vi "2100_Test_Set State_Measure Resistance_SH3T_Rfree_w Config.vi"(0 "Semiconductor Module Context":T7, 1 "Script_Info":T3={"Script Name"="WalkingState", "All_Scripts"=[]}, 4 "Instrument_Pins":T6={"SMU_Pins"=["RF1", "RF2", "RF3", "RF4"], "HSDIO_Pins"=["CLK", "SDA"]}, 5 "Error In":errorcluster, 6 "USID":T4 max=15, 7 "Master_Register_Data_Array_In":T1 {"Address" format="%.0x"}, 8 "current range":dbl format="%#_6p", 10 "current level":dbl=1e-05 format="%#_13p", 11 "Reg_Map_and_Bit_Name":T5={"Reg_Map_Bit_Name"="", "Reg_Map"=[["Reg Addr(0x00)", "7", "6", "5", "4", "3", "2", "1", "0"], ["0", "SPARE", "RF3_SH", "RF2_SH", "RF1_SH", "SPARE", "RF3_RFC", "RF2_RFC", "RF1_RFC"], ["1", "SPARE[7:0]", "", "", "", "", "", "", ""], ["2", "VVAR_EN", "LCM_EN", "RFC_SH", "SPARE", "VARACTOR[3:0]", "", "", ""], ["3", "SW_CTRL1_VIRTUAL[7:0]", "", "", "", "", "", "", ""], ["4", "SW_CTRL1_SWAP", "SW_CTRL1_RBSHIFT[2:0]", "", "", "SW_CTRL1_VSID[3:0]", "", "", ""], ["5", "REG_00_VIRTUAL_MASK[7:0]", "", "", "", "", "", "", ""], ["6", "LOCK_STATUS[1:0]", "", "CLK_DITHER", "FUSES_BURNED", "CLK_IDAC_CAL[3:0]", "", "", ""], ["7", "SPARE[2:0]", "", "", "ODFT_TRIM[4:0]", "", "", "", ""], ["8", "SPARE[2:0]", "", "", "HV_TRIM[4:0]", "", "", "", ""], ["9", "TEST_MUX[2:0]", "", "", "SPARE[1:0]", "", "MEMS_BG_TC[1:0]", "", "MEMSCP_RCM"], ["A", "CP_BOOST_OVRD_EN", "SPARE[2:0]", "", "", "PS_OFF_TIMER[1:0]", "", "PS_ON_TIMER[1:0]", ""], ["0", "", "", "", "", "", "", "", ""], ["D", "Reserved[1:0]", "", "WD_HI_EVENT_CNT[5:0]", "", "", "", "", ""], ["E", "VERSION_ID[7:0]", "", "", "", "", "", "", ""], ["F", "Reserved", "COUNT_200_LSB[6:0]", "", "", "", "", "", ""], ["10", "CLK_DIV2_EN", "Spare", "ODFT_EN", "HV_HYST[4:0]", "", "", "", ""], ["0", "", "", "", "", "", "", "", ""], ["12", "SHORT_FUSE", "FUSE_BURN", "STROBE_EN", "VIO_OK", "RTH[1:0]", "", "FUSE_LOAD_MAN_EN", "FUSE_LOAD"], ["13", "RR_ACK_EN", "Reserved", "ACK_POSITION[1:0]", "", "SuBUS_DRIVE_STRENGTH[3:0]", "", "", ""], ["14", "TM_IO_EN", "TM_IO_SEL", "SuBUS_OVS[1:0]", "", "Reserved[3:0]", "", "", ""], ["15", "Reserved[4:0]", "", "", "", "", "SuBUS_VERSION_PRESENT", "SuBUS_VOLTAGE", "SuBUS_FLAVOR_DEF"], ["16", "PROG_STROBE1_DUR[7:0]", "", "", "", "", "", "", ""], ["17", "PROG_STROBE0_DUR[7:0]", "", "", "", "", "", "", ""], ["18", "Reserved[2:0]", "", "", "EFUSE_SINGLE_ADDR_SEL[4:0]", "", "", "", ""], ["19", "POLL_ADR[4:0]", "", "", "", "", "POLL_BC[2:0]", "", ""], ["1A", "SOFTWARE_RESET", "Reserved[6:0]", "", "", "", "", "", ""], ["1B", "Reserved[7:0]", "", "", "", "", "", "", ""], ["1C", "PWR_MODE_1", "PWR_MODE_0", "TRIGGER_MASK[2:0]", "", "", "TRIGGER[2:0]", "", ""], ["1D", "PRODUCT_ID[7:0]", "", "", "", "", "", "", ""], ["1E", "MANUFACTURER_ID_LSB[7:0]", "", "", "", "", "", "", ""], ["1F", "MANUFACTURER_ID_MSB[3:0]", "", "", "", "USID[3:0]", "", "", ""]]}, 12 "R_Guardian":dbl[](array[numeric])) -> (15 "Master_Register_Data_Array_Out":T1 {"Address" format="%.0x"}, 19 "Error Out":errorcluster)   [LabVIEW 2013]
uses:
  Controls/USID.ctl
  <vilib>/NI_TestStand_SemiconductorModule/NI_TestStand_Semiconductor_Module.lvlibp/PinMap/General/SemiconductorModuleContext.ctl
  Controls/Master_Reg_Data_Array.ctl
  Controls/Reg_Address_Data.ctl
  <vilib>/NI_TestStand_SemiconductorModule/NI_TestStand_Semiconductor_Module.lvlibp/PinMap/General/Publish/PublishDataDoubleFunctionalTest.vi
  <vilib>/NI_TestStand_SemiconductorModule/NI_TestStand_Semiconductor_Module.lvlibp
panel:
  out "Data_Names":string[](array[string])
  out "Logged_Data":dbl[](array[numeric]) format="%#_6p"
  out "R_Measurements":dbl[][](array[numeric]) format="%#_6p"
  in  "Tab Control":enum32{"Test Info", "Instrument Settings"}(tab)
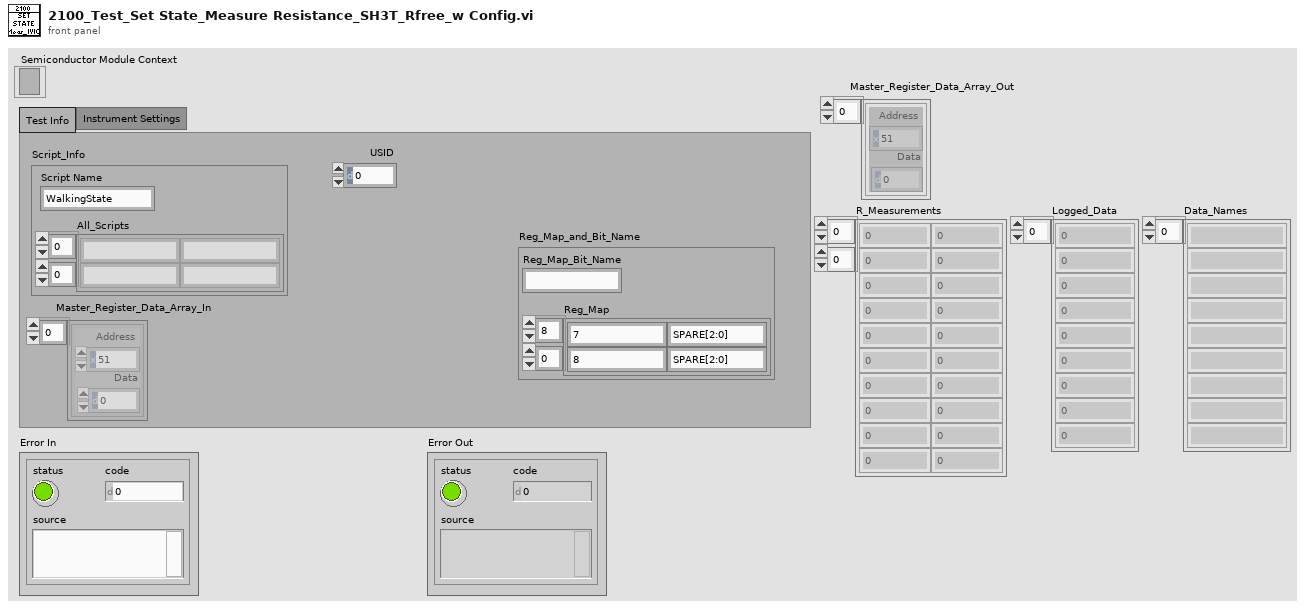
[diagram p1: front panel]
types:
  T1 = typedef "Master_Reg_Data_Array.ctl" = T2[]
  T2 = typedef "Reg_Address_Data.ctl" = cluster{"Address":u8, "Data":u8}
  T3 = cluster{"Script Name":string, "All_Scripts":string[][]}
  T4 = typedef "USID.ctl" = u8
  T5 = cluster{"Reg_Map_Bit_Name":string, "Reg_Map":string[][]}
  T6 = cluster{"SMU_Pins":string[], "HSDIO_Pins":string[]}
  T7 = typedef "NI_TestStand_Semiconductor_Module.lvlibp/SemiconductorModuleContext.ctl" = refnum<k7>
  T8 = typedef "Script Functions_Array.ctl" = enum16{"Reg_Write", "Bit_Write", "Delay", "Read", "Measure"}[]
  T9 = enum16{"Reg_Write", "Bit_Write", "Delay", "Read", "Measure"}
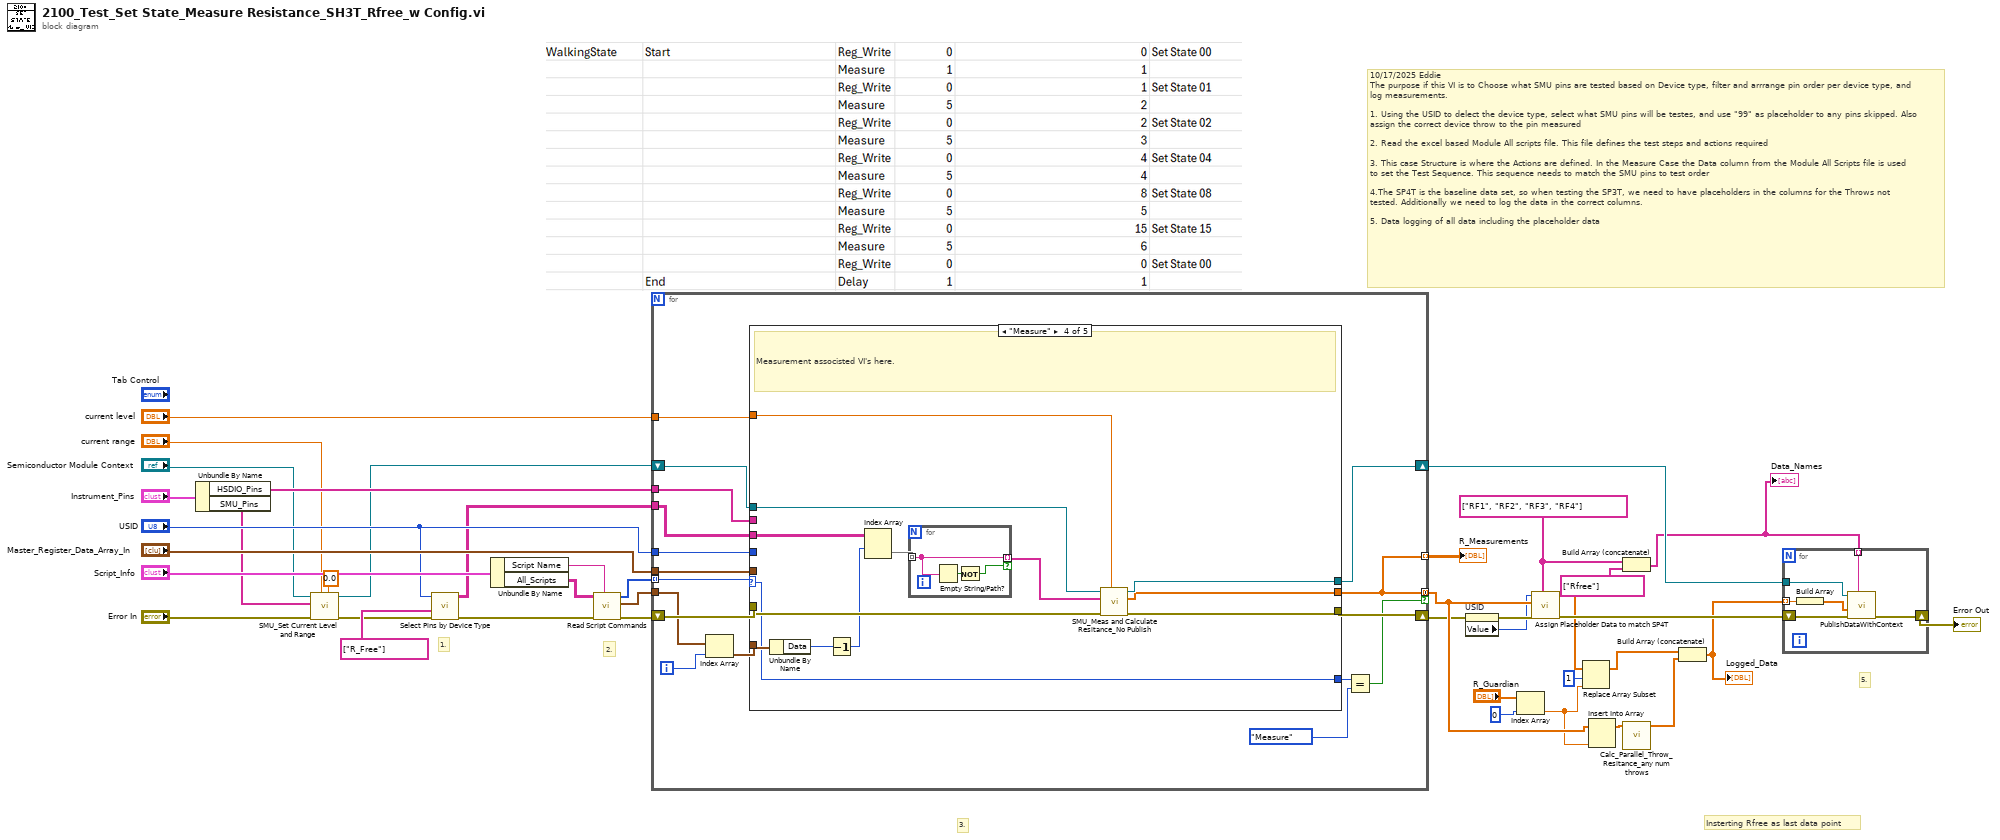
[diagram p0: block diagram]
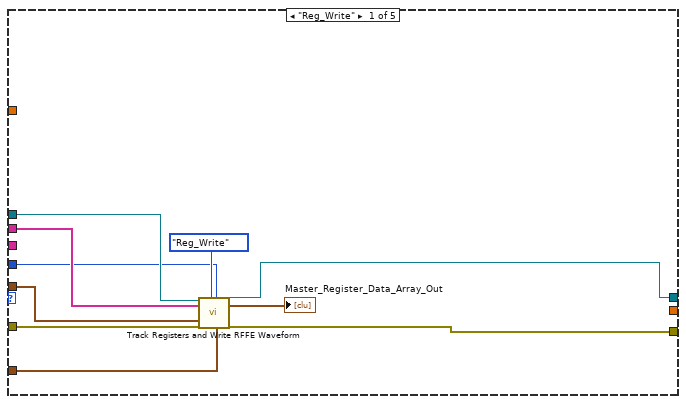
[diagram p2: hidden frame]
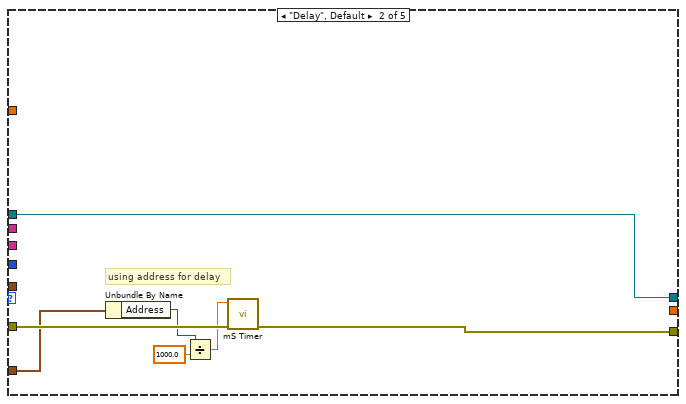
[diagram p3: hidden frame]
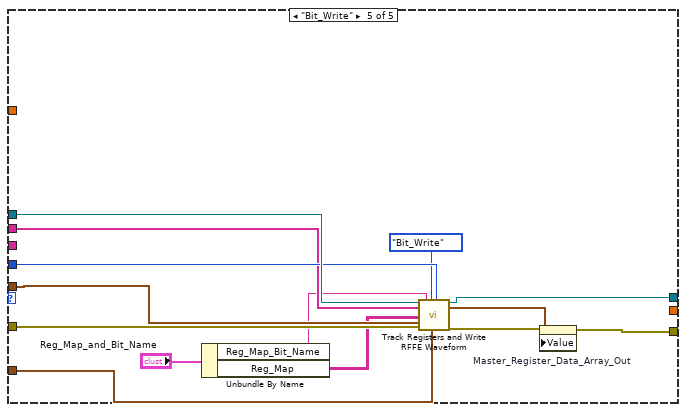
[diagram p5: hidden frame]
diagram:
  w24 = string[] ["RF1", "RF2", "RF3", "RF4"] ("SP4T_Pins")
  # "Insterting Rfree as last data point"
  # "10/17/2025 Eddie \nThe purpose if this VI is to Choose what SMU pins are tested based on Device type, filter and arrrange pin order per device type, and log measurements.\n\n1. Using the USID to delect the device type, select what SMU pins will be testes, and use \"99\" as placeholder to any pins skipped. Also assign the correct device throw to the pin measured\n\n2. Read the excel based Module All scripts file. This file defines the test steps and actions required\n\n3. This case Structure is where the Actions are defined. In the Measure Case the Data column from the Module All Scripts file is used to set the Test Sequence. This sequence needs to match the SMU pins to test order\n\n4.The SP4T is the baseline data set, so when testing the SP3T, we need to have placeholders in the columns for the Throws not tested. Additionally we need to log the data in the correct columns.\n\n5. Data logging of all data including the placeholder data"
  # "5."
  # "3."
  # "2."
  # "1."
  n1 = Unbundle By Name("Instrument_Pins") -> ("HSDIO_Pins"=w35:string[], "SMU_Pins"=w6:string[])
  n2 = call "SMU_Set Current Level and Range.vi"("current level"=0.0, "current range"="current range", "error in (no error)"="Error In", "Pins"=w6, "Semiconductor Module Context"="Semiconductor Module Context") -> ("error out"=w7:errorcluster, "Semiconductor Module Context Out"=w4:T7)  [unwired: 5 in]
  n3 = call "Select Pins by Device Type.vi"("error in (no error)"=w7, "Publishable IDs"=string[] ["R_Free"], "USID"="USID") -> ("error out"=w31:errorcluster, "Pins to Test"=w29:string[][])  [unwired: 7 in]
  n4 = Unbundle By Name("Script_Info") -> ("Script Name"=w32:string, "All_Scripts"=w33:string[][])
  n5 = call "Read Script Commands.vi"("Test Name"=w32, "Error In"=w31, "All_Scripts"=w33) -> ("Error Out"=w39:errorcluster, "Script_Data"=w40:T2[], "Script_Functions"=w41:T8)  [unwired: 5 in, 1 out]
  n6 = for {
    tunnel: "USID" -> [w52]
    tunnel: w41 -> [w51] mode=indexing
    tunnel: w40 -> [w55]
    tunnel: w35 -> [w56]
    shift-right: [w49] -> w11
    shift-left: w39 -> [w58]
    tunnel: "Master_Register_Data_Array_In" -> [w53]
    tunnel: [w47] -> w37 mode=indexing
    tunnel: w29 -> [w48]
    tunnel: [w47] -> w16 mode=concatenating if=w43
    shift-right: [w46] -> w27
    shift-left: w4 -> [w57]
    tunnel: "current level" -> [w42]
    i -> [w50]
    n7 = Index Array(array=w55, index=w50) -> (element=w54:T2)
    n8 = case shown="\"Measure\"" w51 {
      selector: w51 -> [_ _ _ w80 _]
      tunnel: w54 -> [w63 w74 _ w87 w94]
      tunnel: w58 -> [w68 w75 w77 w89 w107]
      tunnel: w52 -> [w60 _ _ _ w101]
      tunnel: w57 -> [w66 w69 w76 w88 w102]
      tunnel: w56 -> [w65 _ _ _ w99]
      tunnel: [w67 w73 w77 w90 w105] -> w49
      tunnel: w53 -> [w62 _ _ _ w98]
      tunnel: [_ _ _ w81 _] -> w47
      tunnel: w48 -> [_ _ _ w86 _]
      tunnel: [w59 w69 w76 w85 w103] -> w46
      tunnel: [_ _ _ w80 _] -> w45
      tunnel: w42 -> [_ _ _ w78 _]
      frame "Reg_Write" {
        n9 = call "Track Registers and Write RFFE Waveform.vi"("Semiconductor Module Context"=w66, "Pins"=w65, "Master_Register_Data_Array_In"=w62, "Error In"=w68, "Script_Functions"=enum16{"Reg_Write", "Bit_Write"}."Reg_Write", "USID"=w60, "Reg_Address_Data"=w63) -> ("Semiconductor Module Context Out"=w59:T7, "Master_Register_Data_Array_Out"=→"Master_Register_Data_Array_Out":T1, "Error Out"=w67:errorcluster)  [unwired: 10 in]
      }
      frame "Delay", Default {
        # "using address for delay"
        n10 = Unbundle By Name(w74) -> ("Address"=w71:u8)
        n11 = Divide(x=w71, y=1000.0) -> (x/y=w70:dbl)
        n12 = call "mS Timer.vi"("Error In"=w75, "Delay(S)"=w70) -> ("Error Out"=w73:errorcluster)  [unwired: 9 in]
      }
      frame "Read" {
        # "Future Dev Code"
      }
      frame "Measure" {
        # "Measurement associsted VI's here."
        n13 = Unbundle By Name(w87) -> ("Data"=w83:u8)
        n14 = Decrement(x=w83) -> (x-1=w82:u8)
        n15 = Index Array(array=w86, index (row)=w82) -> (element=w84:string[])  [unwired: 1 in]
        n16 = for {
          tunnel: w84 -> [w93] mode=indexing
          tunnel: [w93] -> w79 mode=indexing if=w91
          n17 = Empty String/Path?(string/path=w93) -> (empty?=w92:bool)
          n18 = Not(x=w92) -> (.not. x?=w91:bool)
        }
        n19 = call "SMU_Meas and Calculate Resitance_No Publish.vi"("Current  Level"=w78, "error in (no error)"=w89, "Pins"=w79, "Semiconductor Module Context"=w88) -> ("error Out"=w90:errorcluster, "R Array"=w81:dbl[], "Semiconductor Module Context Out"=w85:T7)  [unwired: 4 in, 1 out]
      }
      frame "Bit_Write" {
        n20 = Unbundle By Name("Reg_Map_and_Bit_Name") -> ("Reg_Map_Bit_Name"=w96:string, "Reg_Map"=w95:string[][])
        n21 = call "Track Registers and Write RFFE Waveform.vi"("Semiconductor Module Context"=w102, "Pins"=w99, "Reg_Map"=w95, "Master_Register_Data_Array_In"=w98, "Error In"=w107, "Reg_Map_Bit_Name"=w96, "Script_Functions"=enum16{"Reg_Write", "Bit_Write"}."Bit_Write", "USID"=w101, "Reg_Address_Data"=w94) -> ("Semiconductor Module Context Out"=w103:T7, "Master_Register_Data_Array_Out"=w104:T1, "Error Out"=w106:errorcluster)  [unwired: 8 in]
        n22 = property on="Master_Register_Data_Array_Out" class="Arr (strict)"(error in=w106, "Value"=w104) -> (error out=w105:errorcluster)  [unwired: 1 in, 1 out]
      }
    }
    n23 = Equal?(x=w45, y=T9."Measure" ("Enum")) -> (x = y?=w43:bool)
  }
  "R_Measurements" <- w37
  n24 = property on="USID" class="DigNum (strict)"(error in=w11) -> (error out=w10:errorcluster, "Value"=w9:T4)  [unwired: 1 in, 1 out]
  n25 = Index Array(array="R_Guardian", index=0) -> (element=w15:dbl)
  n26 = call "Assign Placeholder Data to match SP4T.vi"("SP4T_Pins"=w24, "error in (no error)"=w10, "Individual_R_Meas"=w16, "USID"=w9) -> ("error out"=w25:errorcluster, "Placeholder_w_Data"=w19:dbl[])  [unwired: 6 in]
  n27 = Replace Array Subset(array=w19, new element=w15, index=1) -> (w13:dbl[])
  n28 = Insert Into Array(array=w16, new element=w15) -> (w17:dbl[])  [unwired: 1 in]
  n29 = Build Array (concatenate)(w24, string[] ["Rfree"] ("element")) -> (w22:string[])
  "Data_Names" <- w22
  n30 = call "Calc_Parallel_Throw_Resitance_any num throws.vi"("Resitance_Per Site"=w17) -> ("Parallel_Resitance"=w14:dbl[])  [unwired: 10 in]
  n31 = Build Array (concatenate)(w13, w14) -> (w12:dbl[])
  "Logged_Data" <- w12
  n32 = for {
    shift-right: [w113] -> w28
    shift-left: w25 -> [w112]
    tunnel: w27 -> [w111]
    tunnel: w22 -> [w110] mode=indexing
    tunnel: w12 -> [w109] mode=indexing
    n33 = Build Array(w109) -> (w108:dbl[])
    n34 = call-poly <vilib>:"PublishDataWithContext.vi"("Published Data Id"=w110, "error in (no error)"=w112, "Data In"=w108, "Semiconductor Module Context"=w111) -> ("error out"=w113:errorcluster)  [unwired: 6 in, 1 out]
  }
  "Error Out" <- w28
